vi "Dashboard Main.vi"() -> ()   [LabVIEW 2013]
uses:
  <vilib>/event_ctls.llb/eventvkey.ctl
  <vilib>/Rock Robotics/WPI/Dashboard/WPI_DashboardLogging Global.vi
  <vilib>/Utility/config.llb/Write Key (String).vi
  <vilib>/Utility/config.llb/Write Key (I32).vi
  <vilib>/Utility/config.llb/NI_LVConfig.lvlib
panel:
  out "Image Message":string="Timeout in Camera Communications"
  in  "Rec Mode":enum32{"Stop", "Record", "Playback"}(radio)
  in  "Dashboard Tab":T1(tab)
  in  "Camera Settings":T2={"Frame Rate"=30, "Compression"=30, "Size"=1} {"Frame Rate" scale=1.0..30.0; "Size" items=["640x480", "320x240", "160x120"]}
  out "Mode":T3(ring)=enum."Auto Disabled"
  out "Camera IP":string
  in  "DB Camera Config":bool
  out "fps":dbl format="%#.1g"
  out "Mbps":dbl format="%#.1g"
  out "Mbps 2":bool
  out "LED 1":bool
  in  "Slider 1":dbl(slide) scale=0.0..100.0
  in  "Checkbox 2":bool
  in  "Checkbox 1":bool
  in  "Test Slider":dbl(slide) scale=0.0..100.0 scale format="%#_3g"
  in  "On/Off":bool caption="Solenoid"
  in  "Test Name":u16(ring) items=["Select the test to run...", "Example Test", "-------------------------------", "List of tests is built in robot code.", "Replace with your own automated tests."]
  in  "Test Tree":string(tree)
  in  "Motor":cluster{"Value":dbl, "Enable":bool} {"Value" scale=-1.0..1.0 scale format="%#_3g"}
  out "Progress":T4 {"Test Progress" scale=0.0..100.0}
  in  "Rev/Fwd":cluster{"Forward":bool, "Reverse":bool}
  in  "Test Ring":u16(ring) items=["Auto", "Fixed indoor", "Fixed outdoor 1", "Fixed outdoor 2", "Fixed fluorescent 1", "Fixed fluorescent 2", "Hold current"]
  in  "Listbox":i32(listbox)
  out "Tree":string(tree)
  out "Camera Image":T5(plugin-control)
  in  "Enable":bool
  # "Customize by placing controls and indicators here and name to\nmatch Dashboard Variables on robot."
  # "This tab is a great place for autonomous settings and validation.\nCustomize by placing controls and indicators here and name to\nmatch Dashboard Variables on robot."
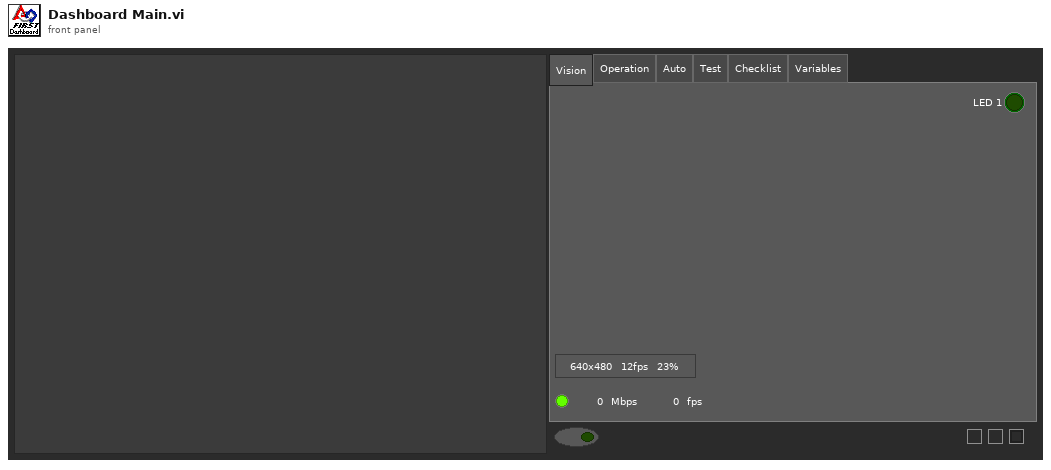
[diagram p1: front panel]
types:
  T1 = enum32{"Vision", "Operation", "Auto", "Test", "Checklist", "Variables"}
  T2 = cluster{"Frame Rate":i32, "Compression":i32, "Size":u16}
  T3 = enum8{"Tele-Op Disabled", "Tele-Op Enabled", "Auto Disabled", "Auto Enabled", "Test Disabled", "Test Enabled", ""}
  T4 = cluster{"Test Progress":u8, "Test Progress Text":string}
  T5 = typedef "IMAQ Image.ctl" = refnum<image>
  T6 = enum32{"Drive", "Operation", "Auto", "Test", "Checklist", "Variables"}
  T7 = typedef "Image Type" = u32
  T8 = cluster{"Digital Inputs":bool[], "Digital Outputs":bool[]}
  T9 = cluster{"Competition mode":bool, "Robot Link":bool, "Autonomous":bool, "Enabled":bool, "E-Stop":bool, "Simulated":bool, "TestMode":bool, "Docked Window":bool}
  T10 = typedef "NI_LVConfig.lvlib/Config Data RefNum.ctl" = refnum<k1>
  T11 = typedef "eventvkey.ctl" = enum16{"ASCII", "Enter", "Return", "Shift", "Ctrl", "Alt", "Cmd", "Opt", "Caps", "NumLock", "Clear", "Break", "Up", "Down", "Left", "Right", "Insert", "Delete", "Home", "End", "PageUp", "PageDown", "Escape", "Help", "Pause", "ScrollLock", "F1", "F2", "F3", "F4", "F5", "F6", "F7", "F8", "F9", "F10", "F11", "F12", "F13", "F14", "F15", "F16", "F17", "F18", "F19", "F20", "F21", "F22", "F23", "F24", "Play", "VolumeUp", "VolumeDown", "Mute", "Two Byte Char"}
  T12 = cluster{"Image Size":bool, "Image Type":bool, "Pixel Value":bool, "ROI Information":bool, "Zoom Factor":bool}
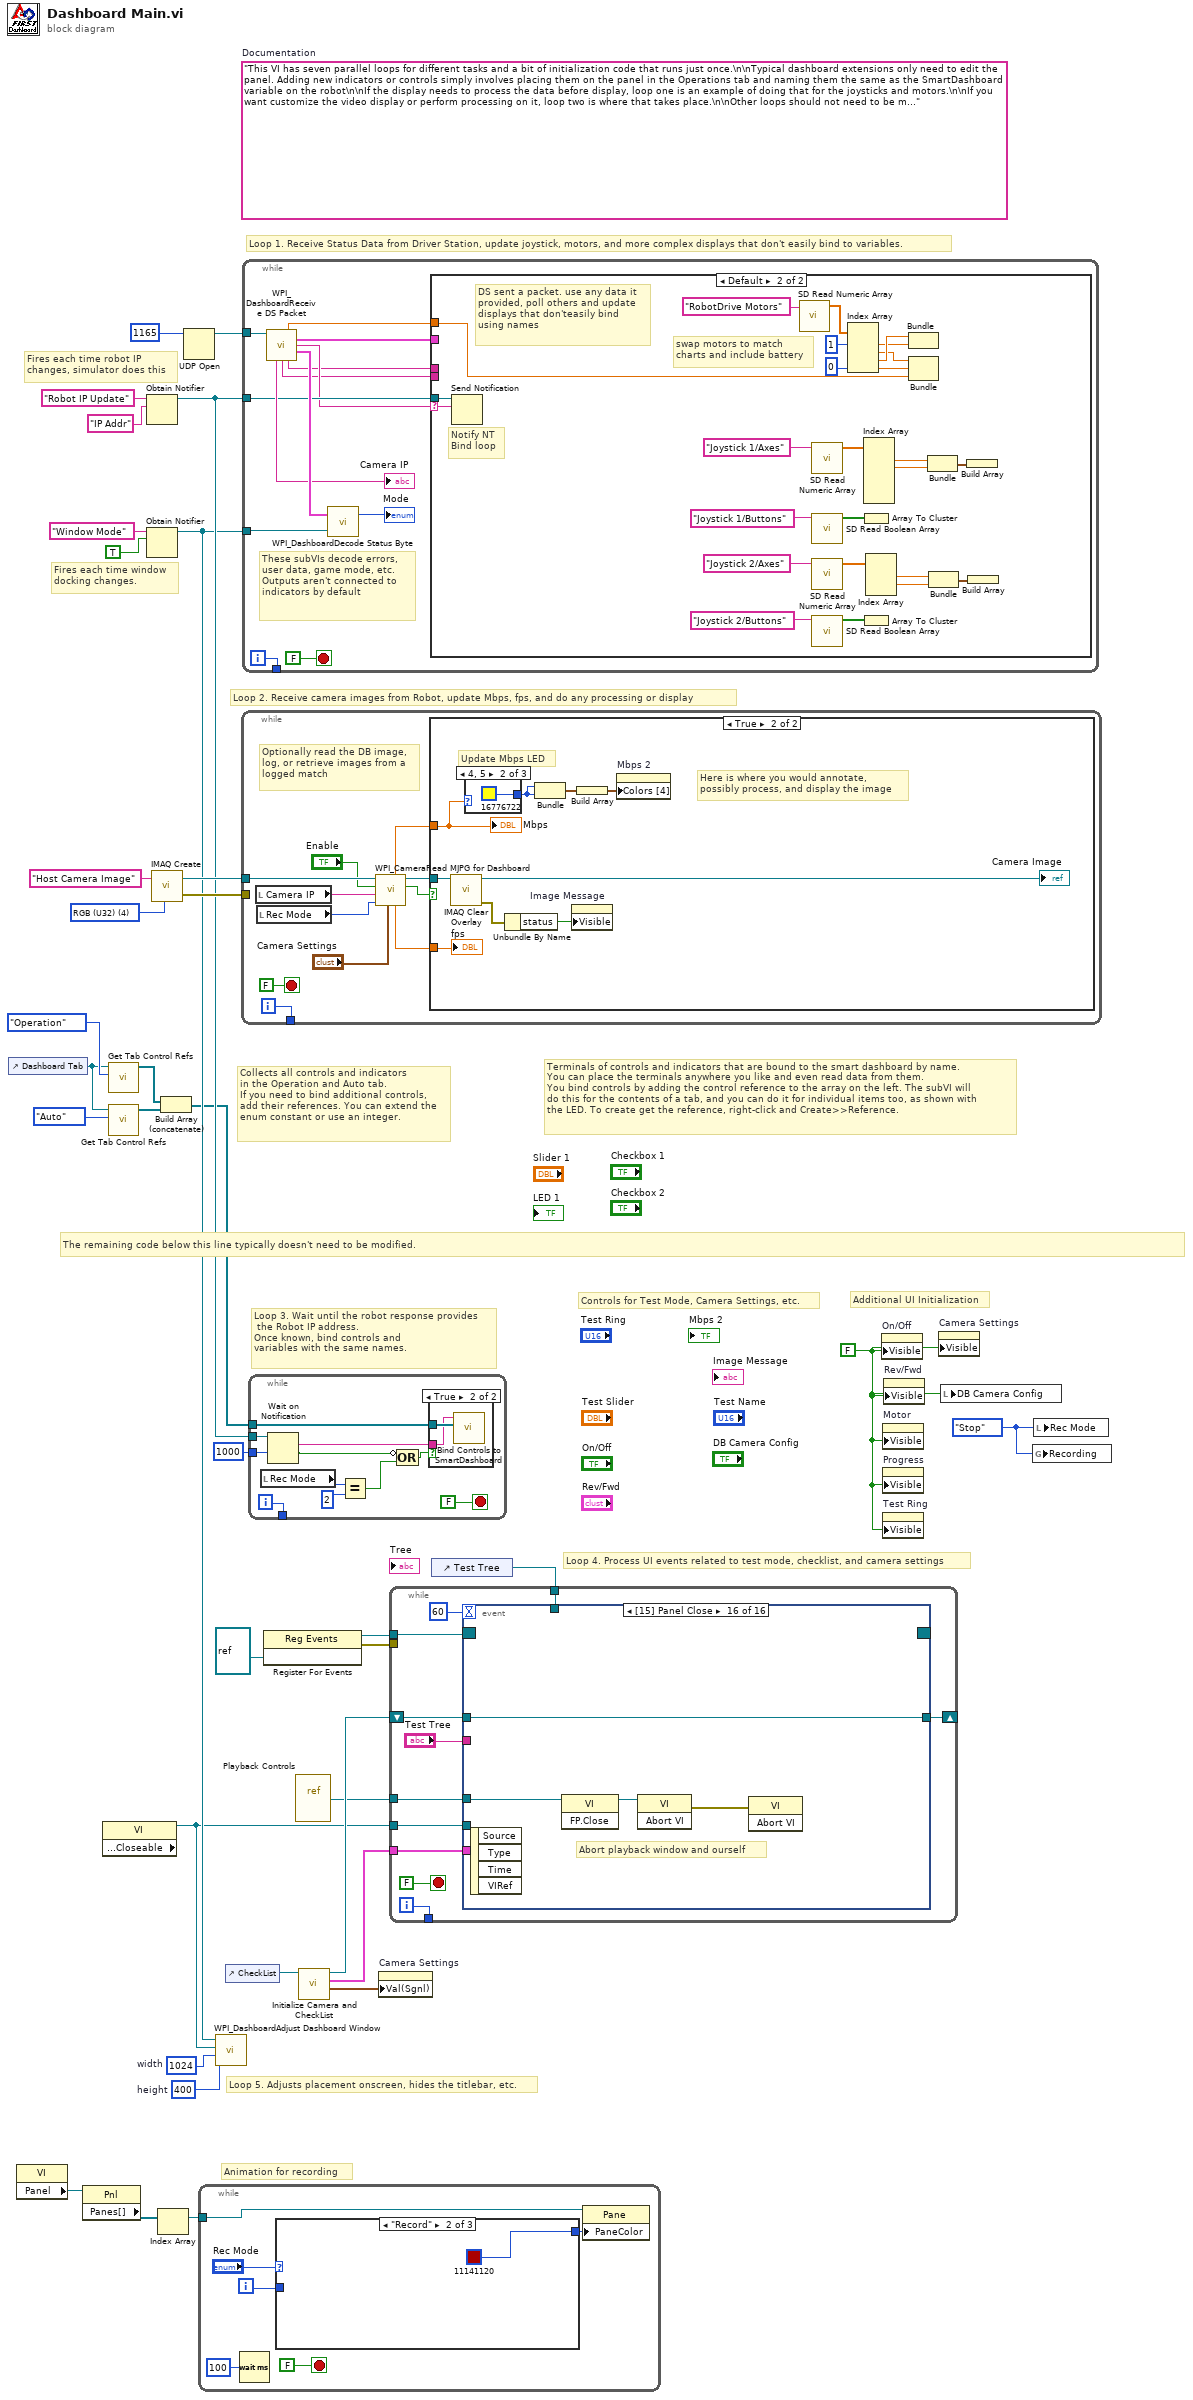
[diagram p0: block diagram]
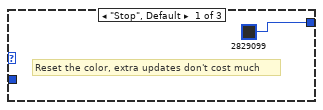
[diagram p2: hidden frame]
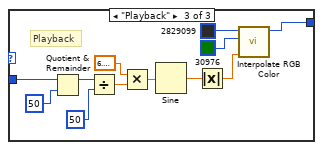
[diagram p3: hidden frame]
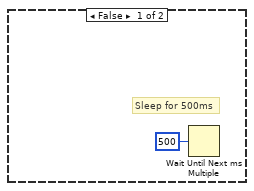
[diagram p5: hidden frame]
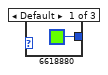
[diagram p6: hidden frame]
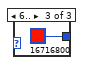
[diagram p7: hidden frame]
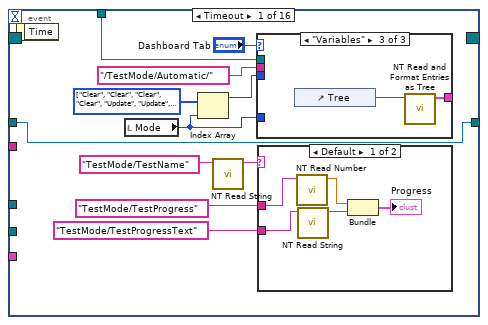
[diagram p8: hidden frame]
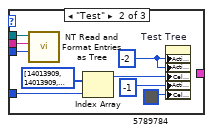
[diagram p10: hidden frame]
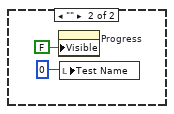
[diagram p11: hidden frame]
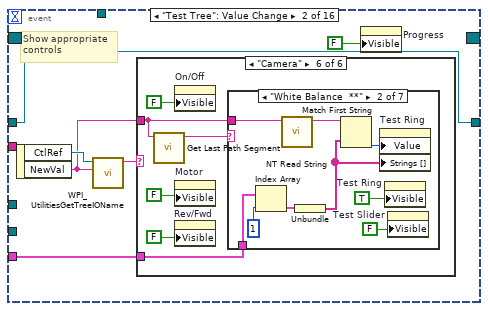
[diagram p12: hidden frame]
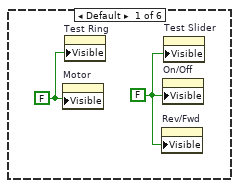
[diagram p13: hidden frame]
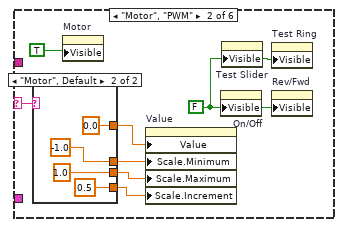
[diagram p14: hidden frame]
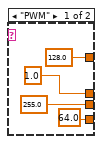
[diagram p15: hidden frame]
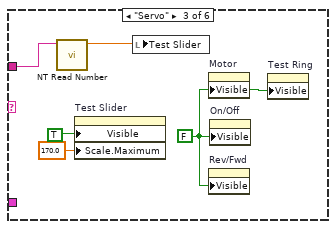
[diagram p16: hidden frame]
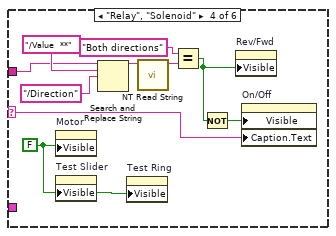
[diagram p17: hidden frame]
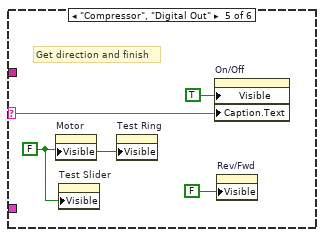
[diagram p18: hidden frame]
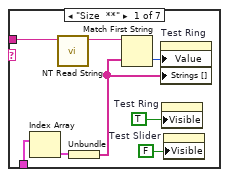
[diagram p19: hidden frame]
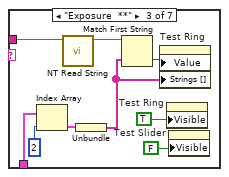
[diagram p20: hidden frame]
diagram:
  w7 = enum32{"Stop", "Record", "Playback"}."Stop" ("Rec Mode")
  w10 = 400  # height
  w11 = 1024  # width
  w24 = FALSE ("Visible")
  (unwired) "This VI has seven parallel loops for different tasks and a bit of initialization code that runs just once.\n\nTypical dashboard extensions only need to edit the panel. Adding new indicators or controls simply involves placing them on the panel in the Operations tab and naming them the same as the SmartDashboard variable on the robot\n\nIf the display needs to process the data before display, loop one is an example of doing that for the joysticks and motors.\n\nIf you want customize the video display or perform processing on it, loop two is where that takes place.\n\nOther loops should not need to be modified. They are pretty standard, and document the task they perform."  # Documentation
  w34 = T7 4 items=["Grayscale (U8)", "Grayscale (I16)", "Grayscale (SGL)", "Complex (CSG)", "RGB (U32)", "HSL (U32)", "RGB (U64)"] ("Image Type")
  # "Controls for Test Mode, Camera Settings, etc."
  # "Additional UI Initialization"
  # "Animation for recording"
  # "Fires each time robot IP\nchanges, simulator does this"
  # "Fires each time window\ndocking changes."
  # "Collects all controls and indicators\nin the Operation and Auto tab.\nIf you need to bind additional controls,\nadd their references. You can extend the\nenum constant or use an integer."
  # "The remaining code below this line typically doesn't need to be modified."
  # "Loop 4. Process UI events related to test mode, checklist, and camera settings"
  # "Terminals of controls and indicators that are bound to the smart dashboard by name.\nYou can place the terminals anywhere you like and even read data from them.\nYou bind controls by adding the control reference to the array on the left. The subVI will\ndo this for the contents of a tab, and you can do it for individual items too, as shown with\nthe LED. To create get the reference, right-click and Create>>Reference."
  # "Loop 3. Wait until the robot response provides\n the Robot IP address.\nOnce known, bind controls and\nvariables with the same names."
  # "Loop 5. Adjusts placement onscreen, hides the titlebar, etc."
  # "Loop 1. Receive Status Data from Driver Station, update joystick, motors, and more complex displays that don't easily bind to variables."
  # "Loop 2. Receive camera images from Robot, update Mbps, fps, and do any processing or display"
  n1 = control-ref of="Dashboard Tab"() -> (w5:refnum<vi>)
  n2 = property class="VI"() -> ("Panel"=w18:refnum<vi>)  [unwired: 2 in, 2 out]
  n3 = property class="Pnl"(reference=w18) -> ("Panes[]"=w19:refnum<vi>[])  [unwired: 1 in, 2 out]
  n4 = property class="VI" props=["Front Panel.Closeable"]() -> (reference out=w6:refnum<vi>)  [unwired: 2 in, 2 out]
  n5 = call <vilib>:"Get Tab Control Refs.vi"("Page Index"=T6."Operation" ("Dashboard Tab"), "TabControl in"=w5) -> ("ControlsOnPage"=w3:refnum<vi>[])  [unwired: 9 in]
  n6 = call <vilib>:"Get Tab Control Refs.vi"("Page Index"=T6."Auto" ("Dashboard Tab"), "TabControl in"=w5) -> ("ControlsOnPage"=w4:refnum<vi>[])  [unwired: 9 in]
  n7 = Obtain Notifier(name (unnamed)="Robot IP Update", notification data type="IP Addr" ("name (unnamed)")) -> (notifier out=w28:refnum<notifier>)  [unwired: 2 in, 2 out]
  n8 = Obtain Notifier(name (unnamed)="Window Mode", notification data type=TRUE) -> (notifier out=w9:refnum<notifier>)  [unwired: 2 in, 2 out]
  n9 = call "IMAQ Create"("Image Name"="Host Camera Image", "Image Type"=w34) -> ("New Image"=w32:T5, "error out"=w31:errorcluster)  [unwired: 2 in, 1 out]
  n10 = Index Array(array=w19) -> (element=w17:refnum<vi>)  [unwired: 1 in]
  n11 = Build Array (concatenate)(w3, w4) -> (w2:refnum<vi>[])
  n12 = UDP Open(11:u16 1165 ("port")) -> (port=w35:refnum<k16>)  [unwired: 2 in, 4 out]
  n13 = while {
    tunnel: w17 -> [w38]
    i -> [w41]
    stop <- FALSE stop-if-true
    n14 = Wait (ms)(milliseconds to wait=u32 100) -> ()  [unwired: 1 out]
    n15 = case shown="\"Record\"" "Rec Mode" {
      tunnel: w41 -> [_ _ w56]
      tunnel: [u32 2829099 ("Base Color") u32 11141120 ("Target Color") w45] -> w37
      frame "Stop", Default {
        # "Reset the color, extra updates don't cost much"
      }
      frame "Record" {
      }
      frame "Playback" {
        # "Playback"
        n16 = Quotient & Remainder(x=w56, y=u32 50 ("milliseconds to wait")) -> (x-y*floor(x/y)=w52:u32)  [unwired: 1 out]
        n17 = Divide(x=w52, y=u32 50 ("milliseconds to wait")) -> (x/y=w49:dbl)
        n18 = Multiply(x=6.283185307179586, y=w49) -> (x*y=w54:dbl)
        n19 = Sine(x=w54) -> (sin(x)=w53:dbl)
        n20 = Absolute Value(x=w53) -> (abs(x)=w46:dbl)
        n21 = call "Interpolate RGB Color.vi"("Proportion"=w46, "Target Color"=u32 30976, "Base Color"=u32 2829099) -> ("Result Color"=w45:u32)  [unwired: 8 in]
      }
    }
    n22 = property class="Pane"(reference=w38, "PaneColor"=w37) -> ()  [unwired: 1 in, 2 out]
  }
  n23 = call <vilib>:"WPI_DashboardAdjust Dashboard Window.vi"("height"=w10, "width"=w11, "reference in"=w6, "Notifier in"=w9) -> ()  [unwired: 8 in]
  n24 = control-ref of="CheckList"() -> (w8:refnum<vi>)
  n25 = while {
    tunnel: w32 -> [w65]
    tunnel: w31 -> [_]
    tunnel: [w66] -> _
    i -> [w66]
    stop <- FALSE stop-if-true
    # "Optionally read the DB image,\nlog, or retrieve images from a\nlogged match"
    n26 = local read "Camera IP"() -> (w58:string)
    n27 = local read "Rec Mode"() -> (w57:enum32{"Stop", "Record", "Playback"})
    n28 = call <vilib>:"WPI_CameraRead MJPG for Dashboard.vi"("Camera Settings"="Camera Settings", "Rec Mode"=w57, "Camera IP"=w58, "Enable"="Enable", "Refnum in"=w65) -> ("Active"=w62:bool, "Refnum out"=w64:T5, "FPS"=w61:dbl, "Bandwidth (Mbps)"=w60:dbl)  [unwired: 3 in]
    n29 = case shown="True" w62 {
      tunnel: w64 -> [_ w72]
      tunnel: w60 -> [_ w71]
      tunnel: w61 -> [_ w69]
      frame False {
        # "Sleep for 500ms"
        n30 = Wait Until Next ms Multiple(millisecond multiple=u32 500) -> ()  [unwired: 1 out]
      }
      frame True {
        # "Here is where you would annotate,\npossibly process, and display the image"
        # "Update Mbps LED"
        n31 = call "IMAQ Clear Overlay"("Image"=w72) -> ("error out"=w76:errorcluster, "Image Out"=→"Camera Image":T5)  [unwired: 2 in, 7 out]
        n32 = case shown="4, 5" w71 {
          tunnel: [u32 6618880 ("Color Box") u32 16776722 ("Color Box") u32 16716800 ("Color Box")] -> w73
          frame Default {
          }
          frame 4, 5 {
          }
          frame 6.. {
          }
        }
        n33 = Unbundle By Name(w76) -> ("status"=w77:bool)
        n34 = Bundle("Color Box"=w73, "Color Box"=w73) -> (w75:cluster{"Color Box":u32, "Color Box":u32})  [unwired: 1 out]
        n35 = property on="Image Message" class="Str"("Visible"=w77) -> ()  [unwired: 2 in, 2 out]
        n36 = Build Array(w75) -> (w74:cluster{"Color Box":u32, "Color Box":u32}[])
        n37 = property on="Mbps 2" class="Bool (strict)"("Colors [4]"=w74) -> ()  [unwired: 2 in, 2 out]
        "Mbps" <- w71
        "fps" <- w69
      }
    }
  }
  n38 = while {
    tunnel: w35 -> [w91]
    tunnel: w28 -> [w86]
    tunnel: w9 -> [w90]
    tunnel: [w87] -> _
    i -> [w87]
    stop <- FALSE stop-if-true
    # "These subVIs decode errors, user data, game mode, etc.\nOutputs aren't connected to indicators by default"
    n39 = call <vilib>:"WPI_DashboardReceive DS Packet.vi"("Recv Socket"=w91) -> ("Battery"=w81:sgl, "Driver Station"=w82:T8, "Robot IP Address"=w85:string, "Status"=w92:T9, "Camera IP Address"=→"Camera IP":string, "Low Priority User Data"=w84:string, "High Priority User Data"=w83:string)  [unwired: 1 in, 7 out]
    n40 = call <vilib>:"WPI_DashboardDecode Status Byte.vi"("Window Mode Notifier"=w90, "Status"=w92) -> ("Mode"=→"Mode":T3)  [unwired: 1 out]
    n41 = case shown="Default" w85 {
      selector: w85 -> [_ w102]
      tunnel: w86 -> [_ w103]
      tunnel: w84 -> [_ _]
      tunnel: w83 -> [_ _]
      tunnel: w82 -> [_ _]
      tunnel: w81 -> [_ w101]
      frame "0.0.0.0" {
        # "DS not sending packets, or no robot exists yet.\nDon't poll the variables"
      }
      frame Default {
        # "Notify NT\nBind loop"
        # "DS sent a packet. use any data it\nprovided, poll others and update\ndisplays that don'teasily bind\nusing names"
        # "swap motors to match\ncharts and include battery"
        n42 = Send Notification(notification=w102, notifier=w103) -> ()  [unwired: 1 in, 2 out]
        n43 = call <vilib>:"SD Read Numeric Array.vi"("Name"="RobotDrive Motors") -> ("Numeric Array"=w100:dbl[])  [unwired: 8 in, 2 out]
        n44 = call <vilib>:"SD Read Numeric Array.vi"("Name"="Joystick 1/Axes") -> ("Numeric Array"=w114:dbl[])  [unwired: 8 in, 2 out]
        n45 = call <vilib>:"SD Read Boolean Array.vi"("Name"="Joystick 1/Buttons") -> ("Boolean Array"=w115:bool[])  [unwired: 8 in, 2 out]
        n46 = call <vilib>:"SD Read Numeric Array.vi"("Name"="Joystick 2/Axes") -> ("Numeric Array"=w110:dbl[])  [unwired: 8 in, 2 out]
        n47 = call <vilib>:"SD Read Boolean Array.vi"("Name"="Joystick 2/Buttons") -> ("Boolean Array"=w109:bool[])  [unwired: 8 in, 2 out]
        n48 = Index Array(array=w100, index #1=1, index #4=0) -> (element #1=w98:dbl, element #2=w97:dbl, element #3=w99:dbl, element #4=w94:dbl)  [unwired: 2 in]
        n49 = Array To Cluster(array=w115) -> ()  [unwired: 1 out]
        n50 = Array To Cluster(array=w109) -> ()  [unwired: 1 out]
        n51 = Index Array(array=w114) -> (element #1=w112:dbl, element #2=w113:dbl)  [unwired: 6 in, 4 out]
        n52 = Index Array(array=w110) -> (element #1=w105:dbl, element #2=w104:dbl)  [unwired: 3 in, 1 out]
        n53 = Bundle("Numeric"=w99, "Numeric"=w98) -> ()  [unwired: 1 in, 1 out]
        n54 = Bundle("Numeric"=w97, "Numeric"=w94, "Battery"=w101) -> ()  [unwired: 1 in, 1 out]
        n55 = Bundle("Numeric"=w112, "Numeric"=w113) -> (w111:cluster{"Numeric":dbl, "Numeric":dbl})  [unwired: 1 in]
        n56 = Bundle("Numeric"=w105, "Numeric"=w104) -> (w106:cluster{"Numeric":dbl, "Numeric":dbl})  [unwired: 1 in]
        n57 = Build Array(w111) -> ()  [unwired: 1 out]
        n58 = Build Array(w106) -> ()  [unwired: 1 out]
      }
    }
  }
  n59 = while {
    tunnel: w2 -> [w129]
    tunnel: w28 -> [w127]
    tunnel: [w125] -> _
    tunnel: u32 1000 ("milliseconds to wait") -> [w124]
    i -> [w125]
    stop <- FALSE stop-if-true
    n60 = local read "Rec Mode"() -> (w120:enum32{"Stop", "Record", "Playback"})
    n61 = Wait on Notification(notifier=w127, timeout in ms (-1)=w124) -> (notification=w126:string, timed out?=w122:bool)  [unwired: 2 in, 2 out]
    n62 = Equal?(x=w120, y=u16 2 ("Rec Mode")) -> (x = y?=w121:bool)
    n63 = Compound Arithmetic op=OR(invert w122, w121) -> (w123:bool)
    n64 = case shown="True" w123 {
      tunnel: w129 -> [_ w131]
      tunnel: w126 -> [_ w130]
      frame False {
      }
      frame True {
        n65 = call <vilib>:"Bind Controls to SmartDashboard.vi"("Bound Control Refs"=w131, "Server IP Address"=w130) -> ()  [unwired: 10 in]
      }
    }
  }
  n66 = register-events(refnum<vi> refnum) -> (reference out=w15:refnum<event-registration>, error out=w14:errorcluster)  [unwired: 2 in]
  n67 = vi-ref "Playback Controls.vi"() -> (w16:refnum<vi>)
  n68 = call "Initialize Camera and CheckList.vi"("ListBox in"=w8) -> ("Cluster"=w22:cluster{"value":i32, "value":i32, "index":i32}, "Array"=w23:cluster{string[]}[], "File Refnum"=w21:T10)  [unwired: 8 in]
  n69 = property on="Camera Settings" class="Clust (strict)"("Val(Sgnl)"=w22) -> ()  [unwired: 2 in, 2 out]
  n70 = control-ref of="Test Tree"() -> (w20:refnum<vi>)
  n71 = while {
    tunnel: w23 -> [w139]
    shift-right: [w138] -> _
    shift-left: w21 -> [w137]
    tunnel: [w136] -> _
    tunnel: w20 -> [w135]
    tunnel: w16 -> [w134]
    tunnel: w15 -> [w133]
    tunnel: w14 -> [_]
    tunnel: w6 -> [w132]
    i -> [w136]
    stop <- FALSE stop-if-true
    n72 = event shown="[15] Panel Close" {
      selector: w133 -> [_ _ _ _ _ _ _ _ _ _ _ _ _ _ _ _]
      dyn-events: [_ _ _ _ _ _ _ _ _ _ _ _ _ w377 _ _] -> _
      timeout: u32 60 ("milliseconds to wait") -> [_ _ _ _ _ _ _ _ _ _ _ _ _ _ _ _]
      tunnel: w135 -> [w149 _ _ _ _ _ _ _ _ _ _ _ _ _ _ _]
      tunnel: "Test Tree" -> [_ _ _ _ _ _ _ _ w346 w354 w356 w360 w368 _ _ _]
      tunnel: w139 -> [_ w173 _ _ _ _ w310 w340 _ _ _ _ _ _ _ _]
      tunnel: [w143 w172 w271 w276 w284 w296 w309 w333 w345 w352 w355 w359 w367 w379 w393 w394] -> w138
      tunnel: w137 -> [w143 w172 w271 w276 w284 w296 w308 w333 w345 w352 w355 w359 w367 w379 w393 w394]
      tunnel: w134 -> [_ _ _ _ _ _ _ _ _ _ _ _ _ w380 _ w397]
      tunnel: w132 -> [_ _ _ _ _ _ _ _ _ _ _ _ _ w375 _ _]
      event Timeout {
        w148 = enum16{"Update", "Clear"}[] [enum."Clear", enum."Clear", enum."Clear", enum."Clear", enum."Update", enum."Update", enum."Clear"] items=["Update", "Clear"]
        n73 = event-data() -> ()  [unwired: 1 in, 1 out]
        n74 = local read "Mode"() -> (w146:T3)
        n75 = Index Array(array=w148, index=w146) -> (element=w147:enum16{"Update", "Clear"})
        n76 = call <vilib>:"NT Read String.vi"("Name"="TestMode/TestName") -> ("String"=w152:string)  [unwired: 9 in, 1 out]
        n77 = case shown="\"Variables\"" "Dashboard Tab" {
          tunnel: w149 -> [_ w162 _]
          tunnel: "/TestMode/Automatic/" ("Name Pattern") -> [_ w161 _]
          tunnel: w147 -> [_ w160 _]
          tunnel: w146 -> [_ w158 _]
          tunnel: [_ _ w164] -> _
          frame "Operation", Default {
          }
          frame "Test" {
            w157 = -2 ("Active Item:Row Number")
            n78 = call <vilib>:"NT Read and Format Entries as Tree.vi"("Operation"=w160, "Name Pattern"=w161, "Tree Refnum"=w162) -> ()  [unwired: 7 in, 2 out]
            n79 = Index Array(array=u32[] [14013909, 14013909, 14013909, 14013909, 14013909, 16777215, 14013909], index=w158) -> (element=w156:u32)
            n80 = property on="Test Tree" class="Tree (strict)"("Active Item Row Number"=w157, "ActiveColNum"=w157, "CellBG"=w156, "Active Item Row Number"=-1 ("Active Item:Row Number"), "CellBG"=u32 5789784 ("Color Box")) -> ()  [unwired: 2 in, 2 out]
          }
          frame "Variables" {
            n81 = control-ref of="Tree"() -> (w163:refnum<vi>)
            n82 = call <vilib>:"NT Read and Format Entries as Tree.vi"("Tree Refnum"=w163) -> ("Formatted Strings"=w164:cluster{"Name":string, "Value":string}[])  [unwired: 9 in, 1 out]
          }
        }
        n83 = case shown="Default" w152 {
          tunnel: "TestMode/TestProgress" ("Name") -> [w166 _]
          tunnel: "TestMode/TestProgressText" ("Name") -> [w165 _]
          frame Default {
            n84 = call <vilib>:"NT Read Number.vi"("Name"=w166) -> ("Numeric"=w167:dbl)  [unwired: 9 in, 1 out]
            n85 = call <vilib>:"NT Read String.vi"("Name"=w165) -> ("String"=w168:string)  [unwired: 9 in, 1 out]
            n86 = Bundle("Numeric"=w167, "String"=w168) -> (→"Progress":cluster{"Numeric":dbl, "String":string})  [unwired: 1 in]
          }
          frame "" {
            n87 = property on="Progress" class="Clust (strict)"("Visible"=FALSE) -> ()  [unwired: 2 in, 2 out]
            n88 = local write "Test Name"(u16 0) -> ()
          }
        }
      }
      event "Test Tree": Value Change {
        # "Show appropriate\ncontrols"
        n89 = event-data() -> ("CtlRef"=w176:refnum<vi>, "NewVal"=w174:string)  [unwired: 1 in]
        n90 = call <vilib>:"WPI_UtilitiesGetTreeIOName.vi"("NewVal"=w174, "TreeControl in"=w176) -> ("I/O Name"=w177:string)  [unwired: 9 in]
        n91 = case shown="\"Camera\"" w177 {
          selector: w177 -> [_ w184 _ w202 w211 _]
          tunnel: w174 -> [_ _ w199 w201 _ w218]
          tunnel: w173 -> [_ _ _ _ _ w217]
          frame Default {
            w179 = FALSE ("Visible")
            w178 = FALSE ("Visible")
            n92 = property on="Motor" class="Clust (strict)"("Visible"=w178) -> ()  [unwired: 2 in, 2 out]
            n93 = property on="Test Ring" class="Ring (strict)"("Visible"=w178) -> ()  [unwired: 2 in, 2 out]
            n94 = property on="Rev/Fwd" class="Clust (strict)"("Visible"=w179) -> ()  [unwired: 2 in, 2 out]
            n95 = property on="On/Off" class="Bool (strict)"("Visible"=w179) -> ()  [unwired: 2 in, 2 out]
            n96 = property on="Test Slider" class="Slide (strict)"("Visible"=w179) -> ()  [unwired: 2 in, 2 out]
          }
          frame "Motor", "PWM" {
            w185 = FALSE ("Visible")
            n97 = case shown="\"Motor\", Default" w184 {
              tunnel: [1.0 ("Value") -1.0 ("Value")] -> w183
              tunnel: [255.0 ("Value") 1.0 ("Value")] -> w182
              tunnel: [128.0 ("Value") 0.0 ("Value")] -> w181
              tunnel: [64.0 ("Value") 0.5 ("Value")] -> w180
              frame "PWM" {
              }
              frame "Motor", Default {
              }
            }
            n98 = property on="Motor" class="Clust (strict)"("Visible"=TRUE) -> ()  [unwired: 2 in, 2 out]
            n99 = property on="Value" class="Slide (strict)"("Value"=w181, "Scale.Minimum"=w183, "Scale.Maximum"=w182, "Scale.Increment"=w180) -> ()  [unwired: 2 in, 2 out]
            n100 = property on="On/Off" class="Bool (strict)"("Visible"=w185) -> ()  [unwired: 2 in, 2 out]
            n101 = property on="Test Slider" class="Slide (strict)"("Visible"=w185) -> ()  [unwired: 2 in, 2 out]
            n102 = property on="Test Ring" class="Ring (strict)"("Visible"=w185) -> ()  [unwired: 2 in, 2 out]
            n103 = property on="Rev/Fwd" class="Clust (strict)"("Visible"=w185) -> ()  [unwired: 2 in, 2 out]
          }
          frame "Servo" {
            w197 = FALSE ("Visible")
            n104 = call <vilib>:"NT Read Number.vi"("Name"=w199) -> ("Numeric"=w198:dbl)  [unwired: 9 in, 1 out]
            n105 = property on="Test Slider" class="Slide (strict)"("Visible"=TRUE, "Scale.Maximum"=170.0 ("Scale.Range:Maximum")) -> ()  [unwired: 2 in, 2 out]
            n106 = local write "Test Slider"(w198) -> ()
            n107 = property on="Motor" class="Clust (strict)"("Visible"=w197) -> ()  [unwired: 2 in, 2 out]
            n108 = property on="Rev/Fwd" class="Clust (strict)"("Visible"=w197) -> ()  [unwired: 2 in, 2 out]
            n109 = property on="On/Off" class="Bool (strict)"("Visible"=w197) -> ()  [unwired: 2 in, 2 out]
            n110 = property on="Test Ring" class="Ring (strict)"("Visible"=w197) -> ()  [unwired: 2 in, 2 out]
          }
          frame "Relay", "Solenoid" {
            w200 = FALSE ("Visible")
            n111 = property on="Motor" class="Clust (strict)"("Visible"=w200) -> ()  [unwired: 2 in, 2 out]
            n112 = property on="Test Slider" class="Slide (strict)"("Visible"=w200) -> ()  [unwired: 2 in, 2 out]
            n113 = Search and Replace String(input string=w201, search string="/Value  **", replace string="/Direction") -> (result string=w207:string)  [unwired: 5 in, 3 out]
            n114 = property on="Test Ring" class="Ring (strict)"("Visible"=w200) -> ()  [unwired: 2 in, 2 out]
            n115 = call <vilib>:"NT Read String.vi"("Name"=w207) -> ("String"=w205:string)  [unwired: 9 in, 1 out]
            n116 = Equal?(x="Both directions", y=w205) -> (x = y?=w203:bool)
            n117 = Not(x=w203) -> (.not. x?=w204:bool)
            n118 = property on="Rev/Fwd" class="Clust (strict)"("Visible"=w203) -> ()  [unwired: 2 in, 2 out]
            n119 = property on="On/Off" class="Bool (strict)"("Visible"=w204, "Caption.Text"=w202) -> ()  [unwired: 2 in, 2 out]
          }
          frame "Compressor", "Digital Out" {
            w210 = FALSE ("Visible")
            # "Get direction and finish"
            n120 = property on="Motor" class="Clust (strict)"("Visible"=w210) -> ()  [unwired: 2 in, 2 out]
            n121 = property on="Test Slider" class="Slide (strict)"("Visible"=w210) -> ()  [unwired: 2 in, 2 out]
            n122 = property on="Test Ring" class="Ring (strict)"("Visible"=w210) -> ()  [unwired: 2 in, 2 out]
            n123 = property on="On/Off" class="Bool (strict)"("Visible"=TRUE, "Caption.Text"=w211) -> ()  [unwired: 2 in, 2 out]
            n124 = property on="Rev/Fwd" class="Clust (strict)"("Visible"=FALSE) -> ()  [unwired: 2 in, 2 out]
          }
          frame "Camera" {
            n125 = call <vilib>:"Get Last Path Segment.vi"("String in"=w218) -> ("String out"=w219:string)  [unwired: 10 in]
            n126 = property on="On/Off" class="Bool (strict)"("Visible"=FALSE) -> ()  [unwired: 2 in, 2 out]
            n127 = property on="Motor" class="Clust (strict)"("Visible"=FALSE) -> ()  [unwired: 2 in, 2 out]
            n128 = property on="Rev/Fwd" class="Clust (strict)"("Visible"=FALSE) -> ()  [unwired: 2 in, 2 out]
            n129 = case shown="\"White Balance  **\"" w219 {
              tunnel: w218 -> [w225 w234 w243 w252 w261 _ w267]
              tunnel: w217 -> [w223 w231 w240 w249 w258 _ _]
              frame "Size  **" {
                n130 = Index Array(array=w223) -> (element=w222:cluster{string[]})  [unwired: 1 in]
                n131 = call <vilib>:"NT Read String.vi"("Name"=w225) -> ("String"=w224:string)  [unwired: 9 in, 1 out]
                n132 = Unbundle(w222) -> (w220:string[])
                n133 = Match First String(2:w220, 3:w224) -> (0:w221:i32)  [unwired: 1 out]
                n134 = property on="Test Ring" class="Ring (strict)"("Value"=w221, "Strings []"=w220) -> ()  [unwired: 2 in, 2 out]
                n135 = property on="Test Ring" class="Ring (strict)"("Visible"=TRUE) -> ()  [unwired: 2 in, 2 out]
                n136 = property on="Test Slider" class="Slide (strict)"("Visible"=FALSE) -> ()  [unwired: 2 in, 2 out]
              }
              frame "White Balance  **" {
                n137 = Index Array(array=w231, index=1) -> (element=w232:cluster{string[]})
                n138 = call <vilib>:"NT Read String.vi"("Name"=w234) -> ("String"=w233:string)  [unwired: 9 in, 1 out]
                n139 = Unbundle(w232) -> (w229:string[])
                n140 = Match First String(2:w229, 3:w233) -> (0:w228:i32)  [unwired: 1 out]
                n141 = property on="Test Ring" class="Ring (strict)"("Value"=w228, "Strings []"=w229) -> ()  [unwired: 2 in, 2 out]
                n142 = property on="Test Ring" class="Ring (strict)"("Visible"=TRUE) -> ()  [unwired: 2 in, 2 out]
                n143 = property on="Test Slider" class="Slide (strict)"("Visible"=FALSE) -> ()  [unwired: 2 in, 2 out]
              }
              frame "Exposure  **" {
                n144 = Index Array(array=w240, index=2) -> (element=w241:cluster{string[]})
                n145 = call <vilib>:"NT Read String.vi"("Name"=w243) -> ("String"=w242:string)  [unwired: 9 in, 1 out]
                n146 = Unbundle(w241) -> (w237:string[])
                n147 = Match First String(2:w237, 3:w242) -> (0:w238:i32)  [unwired: 1 out]
                n148 = property on="Test Ring" class="Ring (strict)"("Value"=w238, "Strings []"=w237) -> ()  [unwired: 2 in, 2 out]
                n149 = property on="Test Ring" class="Ring (strict)"("Visible"=TRUE) -> ()  [unwired: 2 in, 2 out]
                n150 = property on="Test Slider" class="Slide (strict)"("Visible"=FALSE) -> ()  [unwired: 2 in, 2 out]
              }
              frame "Exposure Priority  **" {
                n151 = Index Array(array=w249, index=3) -> (element=w250:cluster{string[]})
                n152 = call <vilib>:"NT Read String.vi"("Name"=w252) -> ("String"=w251:string)  [unwired: 9 in, 1 out]
                n153 = Unbundle(w250) -> (w246:string[])
                n154 = Match First String(2:w246, 3:w251) -> (0:w247:i32)  [unwired: 1 out]
                n155 = property on="Test Ring" class="Ring (strict)"("Value"=w247, "Strings []"=w246) -> ()  [unwired: 2 in, 2 out]
                n156 = property on="Test Ring" class="Ring (strict)"("Visible"=TRUE) -> ()  [unwired: 2 in, 2 out]
                n157 = property on="Test Slider" class="Slide (strict)"("Visible"=FALSE) -> ()  [unwired: 2 in, 2 out]
              }
              frame "Color Enable  **" {
                n158 = Index Array(array=w258, index=4) -> (element=w259:cluster{string[]})
                n159 = call <vilib>:"NT Read String.vi"("Name"=w261) -> ("String"=w260:string)  [unwired: 9 in, 1 out]
                n160 = Unbundle(w259) -> (w255:string[])
                n161 = Match First String(2:w255, 3:w260) -> (0:w256:i32)  [unwired: 1 out]
                n162 = property on="Test Ring" class="Ring (strict)"("Value"=w256, "Strings []"=w255) -> ()  [unwired: 2 in, 2 out]
                n163 = property on="Test Ring" class="Ring (strict)"("Visible"=TRUE) -> ()  [unwired: 2 in, 2 out]
                n164 = property on="Test Slider" class="Slide (strict)"("Visible"=FALSE) -> ()  [unwired: 2 in, 2 out]
              }
              frame Default {
                n165 = property on="Test Ring" class="Ring (strict)"("Visible"=FALSE) -> ()  [unwired: 2 in, 2 out]
                n166 = property on="Test Slider" class="Slide (strict)"("Visible"=FALSE) -> ()  [unwired: 2 in, 2 out]
              }
              frame "Brightness  **", "Color Level  **", "Compression  **", "FPS  **", "Sharpness  **" {
                n167 = call <vilib>:"NT Read Number.vi"("Name"=w267) -> ("Numeric"=w266:dbl)  [unwired: 9 in, 1 out]
                n168 = local write "Test Slider"(w266) -> ()
                n169 = property on="Test Slider" class="Slide (strict)"("Visible"=TRUE, "Scale.Maximum"=100.0 ("Scale.Range:Maximum")) -> ()  [unwired: 2 in, 2 out]
                n170 = property on="Test Ring" class="Ring (strict)"("Visible"=FALSE) -> ()  [unwired: 2 in, 2 out]
              }
            }
          }
        }
        n171 = property on="Progress" class="Clust (strict)"("Visible"=FALSE) -> ()  [unwired: 2 in, 2 out]
      }
      event "Test Name": Mouse Enter {
        # "Populate the ring with the list of tests"
        n172 = event-data() -> ()  [unwired: 1 in, 1 out]
        n173 = call <vilib>:"NT Read String Array.vi"("Name"="TestMode/TestList") -> ("String Array"=w275:string[])  [unwired: 9 in, 1 out]
        n174 = Build Array (concatenate)("Select the test to run...", w275) -> (w274:string[])
        n175 = property on="Test Name" class="Ring (strict)"("Strings []"=w274) -> ()  [unwired: 2 in, 2 out]
      }
      event "Test Name": Value Change {
        w277 = FALSE ("Visible")
        # "Tell the robot the test name to run"
        n176 = event-data() -> ("NewVal"=w281:u16)  [unwired: 1 in]
        n177 = property on="Test Name" class="Ring (strict)"() -> ("Strings []"=w282:string[])  [unwired: 2 in, 2 out]
        n178 = local write "Progress"(T4 {"Test Progress"=0, "Test Progress Text"=""} ("Progress")) -> ()
        n179 = Index Array(array=w282, index=w281) -> (element=w280:string)
        n180 = call <vilib>:"NT Write String.vi"("String"=w280, "Name"="TestMode/TestName") -> ()  [unwired: 9 in, 1 out]
        n181 = property on="Progress" class="Clust (strict)"("Visible"=TRUE) -> ()  [unwired: 2 in, 2 out]
        n182 = property on="Motor" class="Clust (strict)"("Visible"=w277) -> ()  [unwired: 2 in, 2 out]
        n183 = property on="Test Slider" class="Slide (strict)"("Visible"=w277) -> ()  [unwired: 2 in, 2 out]
        n184 = property on="On/Off" class="Bool (strict)"("Visible"=w277) -> ()  [unwired: 2 in, 2 out]
        n185 = property on="Rev/Fwd" class="Clust (strict)"("Visible"=w277) -> ()  [unwired: 2 in, 2 out]
        n186 = property on="Test Ring" class="Ring (strict)"("Visible"=w277) -> ()  [unwired: 2 in, 2 out]
      }
      event "Listbox": Double Click {
        n187 = event-data() -> ("PlatMods.Shift"=w285:bool, "Row"=w287:i32)  [unwired: 1 in]
        n188 = case shown="True" w285 {
          tunnel: w287 -> [w291 _]
          tunnel: 1 -> [w290 _]
          frame False {
            n189 = property on="Listbox" class="LstBox (strict)"() -> ("Item Symbols"=w289:i32[])  [unwired: 2 in, 2 out]
            n190 = Replace Array Subset(array=w289, new element=w290, index=w291) -> (w288:i32[])
            n191 = property on="Listbox" class="LstBox (strict)"("Item Symbols"=w288) -> ()  [unwired: 2 in, 2 out]
          }
          frame True {
            w292 = 0 ("Top Row")
            n192 = property on="Listbox" class="LstBox (strict)"() -> ("Number of Rows"=w294:u32)  [unwired: 2 in, 2 out]
            n193 = Initialize Array(0, w294) -> (w293:i32[])
            n194 = property on="Listbox" class="LstBox (strict)"("Top Row"=w292, "Value"=w292, "Item Symbols"=w293) -> ()  [unwired: 2 in, 2 out]
          }
        }
      }
      event "Listbox": Key Down {
        n195 = event-data() -> ("VKey"=w298:T11)  [unwired: 1 in]
        n196 = case shown="\"Left\", \"Right\"" w298 {
          selector: w298 -> [w303 _]
          tunnel: eventvkey."Left" ("VKey") -> [w301 _]
          frame "Left", "Right" {
            n197 = Equal?(x=w301, y=w303) -> (x = y?=w302:bool)
            n198 = Select(t=0, s=w302, f=1) -> (s? t:f=w304:i32)
            n199 = property on="Listbox" class="LstBox (strict)"() -> ("Item Symbols"=w307:i32[])  [unwired: 2 in, 2 out]
            n200 = Replace Array Subset(array=w307, new element=w304, index="Listbox") -> (w306:i32[])
            n201 = property on="Listbox" class="LstBox (strict)"("Item Symbols"=w306) -> ()  [unwired: 2 in, 2 out]
          }
          frame Default {
          }
        }
      }
      event "DB Camera Config": Value Change {
        n202 = event-data() -> ("NewVal"=w311:bool)  [unwired: 1 in]
        n203 = case shown="False" w311 {
          tunnel: w310 -> [w320 _]
          tunnel: [w313 w331] -> w309
          tunnel: w308 -> [w312 w331]
          frame False {
            w327 = "Camera"
            w330 = FALSE ("Visible")
            n204 = local read "Camera Settings"() -> (w319:T2)
            n205 = Index Array(array=w320) -> (element=w323:cluster{string[]})  [unwired: 1 in]
            n206 = Unbundle(w319) -> ("Frame Rate"=w318:i32, "Compression"=w317:i32, "Size"=w321:u16)
            n207 = Unbundle(w323) -> (w322:string[])
            n208 = Index Array(array=w322, index=w321) -> (element=w316:string)
            n209 = call-poly <vilib>:"Write Key.vi"("section"=w327, "value"=w316, "key"="Size", "refnum"=w312) -> ("refnum out"=w329:T10)  [unwired: 2 in, 5 out]
            n210 = call-poly <vilib>:"Write Key.vi"("section"=w327, "value"=w318, "key"="FrameRate", "refnum"=w329) -> ("refnum out"=w328:T10)  [unwired: 1 in, 6 out]
            n211 = property on="Camera Settings" class="Clust (strict)"("Visible"=w330) -> ()  [unwired: 2 in, 2 out]
            n212 = local write "DB Camera Config"(w330) -> ()
            n213 = call-poly <vilib>:"Write Key.vi"("section"=w327, "value"=w317, "key"="Compression", "refnum"=w328) -> ("refnum out"=w314:T10)  [unwired: 1 in, 6 out]
            n214 = call <vilib>:"Close Config Data.vi"("refnum"=w314) -> ("file path"=w315:path)  [unwired: 2 in, 8 out]
            n215 = call <vilib>:"Open Config Data.vi"("configuration file path"=w315) -> ("refnum"=w313:T10)  [unwired: 8 in, 2 out]
          }
          frame True {
            n216 = property on="Camera Settings" class="Clust (strict)"("Visible"=TRUE) -> ()  [unwired: 2 in, 2 out]
          }
        }
      }
      event "Camera Settings": Value Change {
        n217 = event-data() -> ("NewVal"=w344:T2)  [unwired: 1 in]
        n218 = Index Array(array=w340) -> (element=w339:cluster{string[]})  [unwired: 1 in]
        n219 = Unbundle(w344) -> ("Frame Rate"=w335:i32, "Compression"=w334:i32, "Size"=w337:u16)
        n220 = Unbundle(w339) -> (w338:string[])
        n221 = Index Array(array=w338, index=w337) -> (element=w336:string)
        n222 = Format Into String(format string="%s   %dfps   %d%%", w336, w335, w334) -> (resulting string=w341:string)  [unwired: 2 in, 1 out]
        n223 = Build Array(w341) -> (w342:string[])
        n224 = property on="DB Camera Config" class="Bool (strict)"("Strings [4]"=w342) -> ()  [unwired: 2 in, 2 out]
      }
      event "Motor.Enable": Value Change {
        n225 = event-data() -> ("NewVal"=w350:bool)  [unwired: 1 in]
        n226 = Unbundle("Motor") -> ("Value"=w349:dbl)  [unwired: 1 out]
        n227 = Select(t=w349, s=w350, f=0.0) -> (s? t:f=w347:dbl)
        n228 = call <vilib>:"NT Write Number.vi"("Numeric"=w347, "Name"=w346) -> ()  [unwired: 9 in, 1 out]
      }
      event "Test Slider": Value Change {
        n229 = event-data() -> ("NewVal"=w353:dbl)  [unwired: 1 in]
        n230 = call <vilib>:"NT Write Number.vi"("Numeric"=w353, "Name"=w354) -> ()  [unwired: 9 in, 1 out]
      }
      event "On/Off": Value Change {
        n231 = event-data() -> ("NewVal"=w358:bool)  [unwired: 1 in]
        n232 = Boolean To (0,1)(Boolean=w358) -> (0, 1=w357:i16)
        n233 = call <vilib>:"NT Write Number.vi"("Numeric"=w357, "Name"=w356) -> ()  [unwired: 9 in, 1 out]
      }
      event "Rev/Fwd": Value Change {
        n234 = event-data() -> ("NewVal.Forward"=w366:bool, "NewVal.Reverse"=w365:bool)  [unwired: 1 in]
        n235 = Boolean To (0,1)(Boolean=w366) -> (0, 1=w362:i16)
        n236 = Boolean To (0,1)(Boolean=w365) -> (0, 1=w364:i16)
        n237 = Negate(x=w364) -> (-x=w363:i16)
        n238 = Add(x=w362, y=w363) -> (x+y=w361:i16)
        n239 = call <vilib>:"NT Write Number.vi"("Numeric"=w361, "Name"=w360) -> ()  [unwired: 9 in, 1 out]
      }
      event "Test Ring": Value Change {
        n240 = event-data() -> ("NewVal"=w370:u16)  [unwired: 1 in]
        n241 = property on="Test Ring" class="Ring (strict)"() -> ("Strings []"=w371:string[])  [unwired: 2 in, 2 out]
        n242 = Index Array(array=w371, index=w370) -> (element=w369:string)
        n243 = call <vilib>:"NT Write String.vi"("String"=w369, "Name"=w368) -> ()  [unwired: 9 in, 1 out]
      }
      event "Rec Mode": Value Change {
        # "Update globals for recording mode and path to read log from.\nClear when logging and let NetworkTables set path for vision to\nuse."
        n244 = event-data() -> ("NewVal"=w381:enum32{"Stop", "Record", "Playback"})  [unwired: 1 in]
        n245 = global write "WPI_DashboardLogging Global.vi" "Logging Filename"(path "") -> ()
        n246 = case shown="\"Stop\", \"Record\"" w381 {
          tunnel: w380 -> [_ w383 w391]
          tunnel: [_ _ w390] -> w377
          tunnel: [_ _ w389] -> _
          tunnel: w375 -> [_ _ w387]
          tunnel: cluster{i32, i32} {-250, 170} -> [_ _ w386]
          tunnel: [_ _ T12 {"Image Size"=TRUE, "Image Type"=TRUE, "Pixel Value"=TRUE, "ROI Information"=TRUE, "Zoom Factor"=FALSE} ("Image Information Shown:All Elements")] -> w373
          tunnel: [_ _ TRUE ("Zoom Factor")] -> w372
          frame Default {
          }
          frame "Stop", "Record" {
            # "Place Window too"
            n247 = invoke class="VI" method="FP.Close"(reference=w383) -> (reference out=w382:refnum<vi>)  [unwired: 2 in, 2 out]
            n248 = invoke class="VI" method="Abort VI"(reference=w382) -> ()  [unwired: 2 in, 3 out]
          }
          frame "Playback" {
            n249 = call "Open Playback Panel.vi"("Offset"=w386, "DB VI Ref"=w387, "Playback in"=w391) -> ("Playback out"=w388:refnum<vi>)  [unwired: 8 in]
            n250 = register-events(w388) -> (reference out=w390:refnum<event-registration>, error out=w389:errorcluster)  [unwired: 2 in]
          }
        }
        n251 = global write "WPI_DashboardLogging Global.vi" "Recording"(w381) -> ()
        n252 = property on="Camera Image" class="ImageControl"("Image Information Shown"=w373, "Image Information Visible"=w372) -> ()  [unwired: 2 in, 2 out]
        n253 = call <vilib>:"WPI_DashboardNT Log FieldName Cache.vi"("Operation"=enum16{"Lookup/Add", "Index", "Clear"}."Clear") -> ()  [unwired: 8 in, 3 out]
      }
      event Panel Close {
        w392 = enum32{"Stop", "Record", "Playback"}."Stop" ("Rec Mode")
        n254 = event-data() -> ()  [unwired: 1 in, 4 out]
        n255 = local write "Rec Mode"(w392) -> ()
        n256 = global write "WPI_DashboardLogging Global.vi" "Recording"(w392) -> ()
      }
      event Panel Close {
        # "Abort playback window and ourself"
        n257 = event-data() -> ()  [unwired: 1 in, 4 out]
        n258 = invoke class="VI" method="FP.Close"(reference=w397) -> (reference out=w396:refnum<vi>)  [unwired: 2 in, 2 out]
        n259 = invoke class="VI" method="Abort VI"(reference=w396) -> (error out=w395:errorcluster)  [unwired: 2 in, 2 out]
        n260 = invoke class="VI" method="Abort VI"(error in=w395) -> ()  [unwired: 2 in, 3 out]
      }
    }
  }
  n261 = property on="On/Off" class="Bool (strict)"("Visible"=w24) -> ()  [unwired: 2 in, 2 out]
  n262 = property on="Motor" class="Clust (strict)"("Visible"=w24) -> ()  [unwired: 2 in, 2 out]
  n263 = property on="Progress" class="Clust (strict)"("Visible"=w24) -> ()  [unwired: 2 in, 2 out]
  n264 = property on="Test Ring" class="Ring (strict)"("Visible"=w24) -> ()  [unwired: 2 in, 2 out]
  n265 = property on="Rev/Fwd" class="Clust (strict)"("Visible"=w24) -> ()  [unwired: 2 in, 2 out]
  n266 = property on="Camera Settings" class="Clust (strict)"("Visible"=w24) -> ()  [unwired: 2 in, 2 out]
  n267 = local write "DB Camera Config"(w24) -> ()
  n268 = global write "WPI_DashboardLogging Global.vi" "Recording"(w7) -> ()
  n269 = local write "Rec Mode"(w7) -> ()
